vi "Initialise.vi"(0 "X":dbl, 5 "Y":dbl, 7 "Facing":dbl, 9 "Size":dbl, 11 "error in (no error)":errorcluster) -> (4 "Car.lvclass":refnum<class "Car.lvclass">, 15 "error out":errorcluster)   [LabVIEW 2015, in "Car.lvclass"]
uses:
  Car.lvclass
  Car.lvclass/Car.ctl
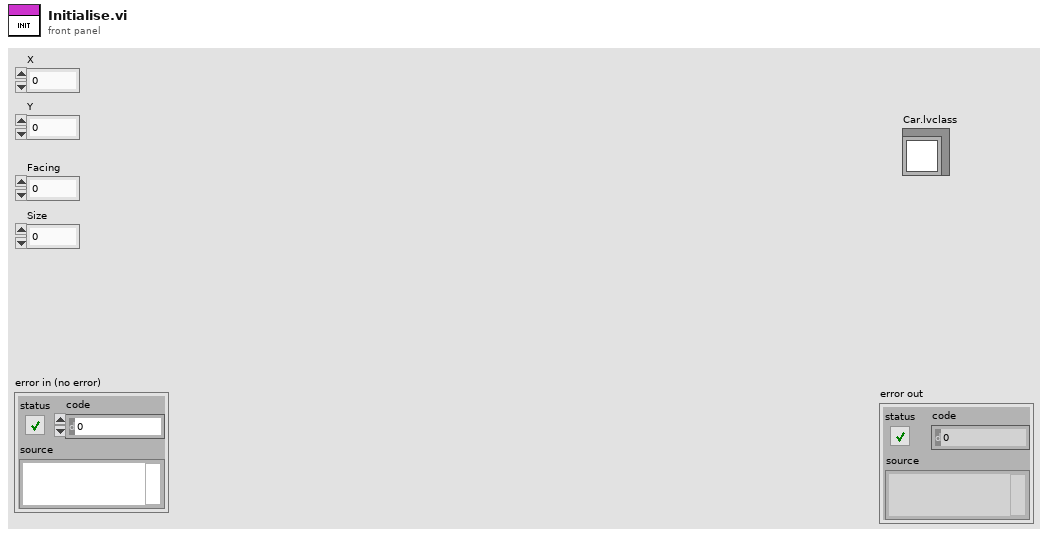
[diagram p1: front panel]
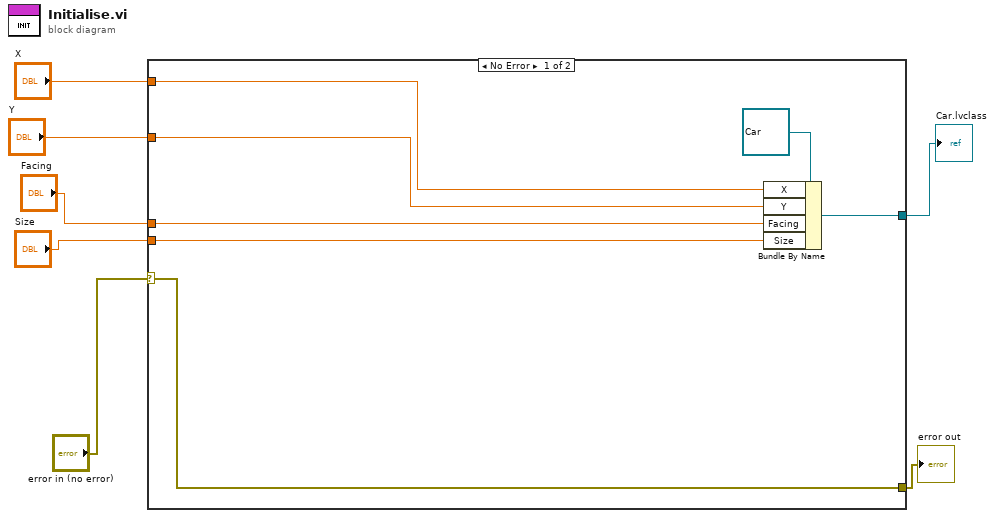
[diagram p0: block diagram]
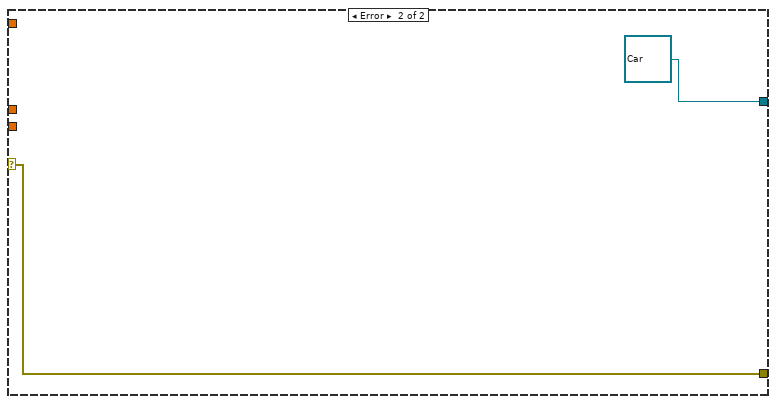
[diagram p2: hidden frame]
diagram:
  n1 = case shown="No Error" "error in (no error)" {
    selector: "error in (no error)" -> [w14 w16]
    tunnel: [w14 w16] -> w6
    tunnel: "X" -> [w12 _]
    tunnel: "Y" -> [w11 _]
    tunnel: "Facing" -> [w10 _]
    tunnel: "Size" -> [w9 _]
    tunnel: [w8 refnum<class "Car.lvclass"> refnum ("Car.lvclass")] -> w1
    frame No Error {
      n2 = Bundle By Name(cluster=refnum<class "Car.lvclass"> refnum ("Car.lvclass"), "X"=w12, "Y"=w11, "Facing"=w10, "Size"=w9) -> (w8:refnum<class "Car.lvclass">)
    }
    frame Error {
    }
  }
  "error out" <- w6
  "Car.lvclass" <- w1
